vi "Tone-Create (cluster).vi"(8 "error in (no error)":errorcluster, 9 "Npts":i32, 10 "Sampling Rate (Hz)":dbl, 11 "Tone Class in":T1) -> (0 "error out":errorcluster, 2 "Waveform":dbl[](array[numeric]), 3 "Tone Class out":T1)   [LabVIEW 2020]
uses:
  Tone Params.ctl
  <vilib>/Analysis/NI_AALBase.lvlib
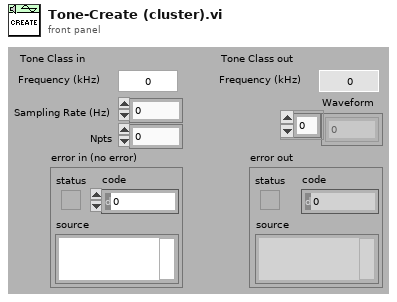
[diagram p1: front panel]
types:
  T1 = typedef "Tone Params.ctl" = cluster{"Frequency (kHz)":dbl, "Last Freq":dbl, "Last Phase":dbl}
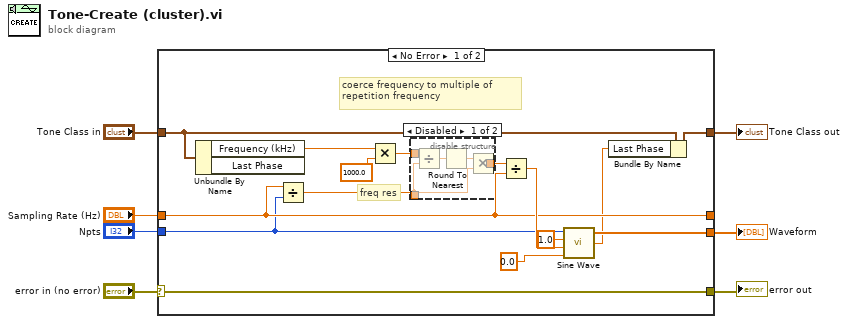
[diagram p0: block diagram]
diagram:
  n1 = case shown="No Error" "error in (no error)" {
    selector: "error in (no error)" -> [w22 w31]
    tunnel: [w22 w31] -> w6
    tunnel: [w10 w30] -> w4
    tunnel: "Tone Class in" -> [w21 w30]
    tunnel: "Npts" -> [w16 _]
    tunnel: "Sampling Rate (Hz)" -> [w17 w29]
    tunnel: [w18 _] -> w1
    tunnel: [w17 w29] -> _
    frame No Error {
      # "freq res"
      # "coerce frequency to multiple of repetition frequency"
      n2 = Unbundle By Name(w21) -> ("Frequency (kHz)"=w11:dbl)  [unwired: 1 out]
      n3 = Divide(x=w17, y=w16) -> (x/y=w15:dbl)
      n4 = Multiply(x=w11, y=1000.0) -> (x*y=w13:dbl)
      n5 = disable-structure shown="Disabled" {
        disable-tunnel: w15 -> [w25 _]
        disable-tunnel: [w24 w28] -> w14
        disable-tunnel: w13 -> [w23 w28]
        frame Disabled {
          n6 = Divide(x=w23, y=w25) -> (x/y=w27:dbl)
          n7 = Round To Nearest(number=w27) -> (nearest integer value=w26:dbl)
          n8 = Multiply(x=w26, y=w25) -> (x*y=w24:dbl)
        }
        frame Enabled {
        }
      }
      n9 = Divide(x=w14, y=w17) -> (x/y=w19:dbl)
      n10 = call <vilib>:"Sine Wave.vi"("samples"=w16, "amplitude"=1.0, "frequency"=w19, "phase in"=0.0) -> ("sine wave"=w18:dbl[], "phase out"=w9:dbl)  [unwired: 1 in, 1 out]
      n11 = Bundle By Name(cluster=w21, "Last Phase"=w9) -> (w10:T1)
    }
    frame Error {
    }
  }
  "error out" <- w6
  "Tone Class out" <- w4
  "Waveform" <- w1
